vi "WaveformChartGraph.vi"() -> ()   [LabVIEW 2018]
panel:
  in  "OK Button":bool
  out "Array":dbl[](array[numeric])
  out "Waveform Graph":dbl[](graph)
  out "Waveform Chart":dbl(graph)
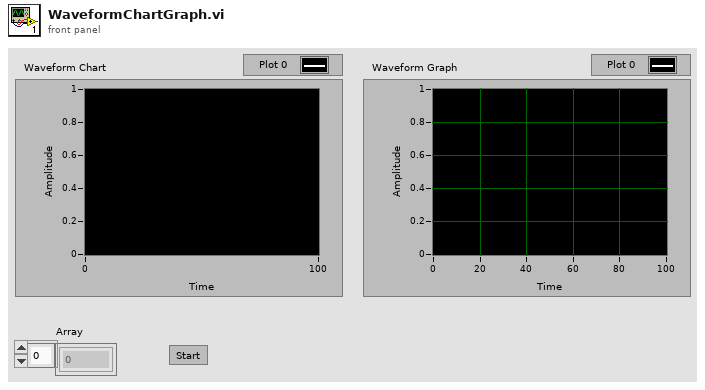
[diagram p1: front panel]
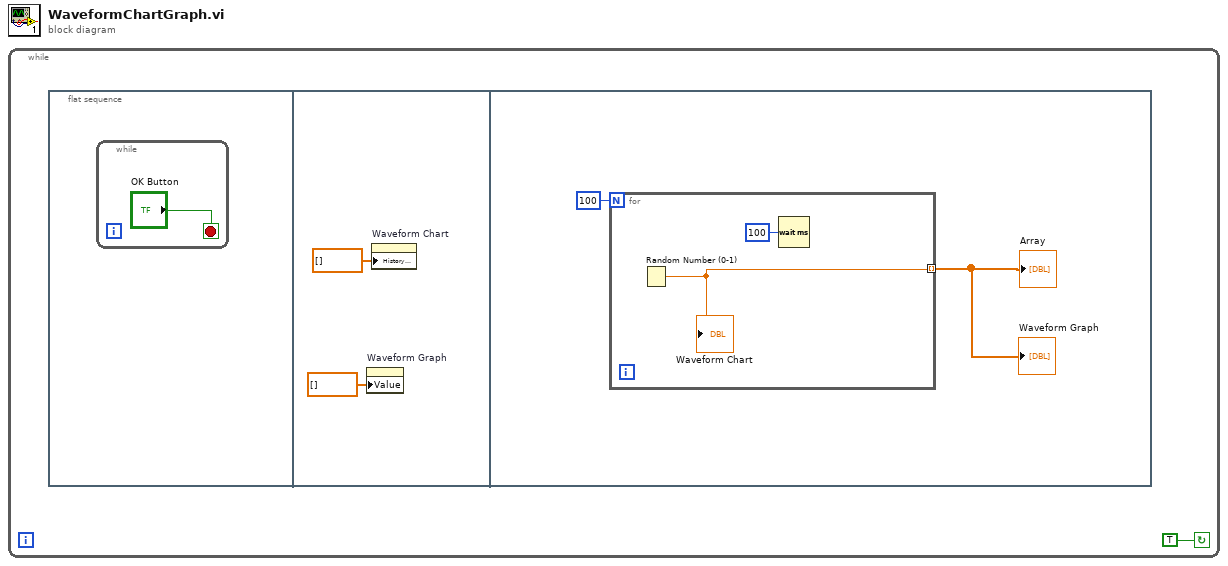
[diagram p0: block diagram]
diagram:
  n1 = while {
    stop <- TRUE continue-if-true
    n2 = flat-sequence {
      frame #0 {
        n3 = while {
          stop <- "OK Button" stop-if-true
        }
      }
      frame #1 {
        n4 = property on="Waveform Graph" class="WFGraph (strict)"("Value"=dbl[] [] ("Waveform Graph")) -> ()  [unwired: 2 in, 2 out]
        n5 = property on="Waveform Chart" class="WFChart (strict)"("History Data"=dbl[] []) -> ()  [unwired: 2 in, 2 out]
      }
      frame #2 {
        n6 = for {
          N: 100 -> [_]
          tunnel: [w8] -> w6 mode=indexing
          n7 = Random Number (0-1)() -> (number: 0 to 1=w8:dbl)
          "Waveform Chart" <- w8
          n8 = Wait (ms)(milliseconds to wait=u32 100) -> ()  [unwired: 1 out]
        }
        "Waveform Graph" <- w6
        "Array" <- w6
      }
    }
  }
